vi "Configure IO Port.vi"(0 "VISA resource name":refnum<visa-resource-name>, 1 "Digital Output Pattern (1111)":u32=15 max=15 format="%04b", 2 "Enable I/O Port Auto Clear (F: Disable)":bool, 5 "Output Line 4 Mode (0: End of Test)":u16(ring) items=["End of Test", "Busy"], 7 "Active TTL Busy Level (0: Active Low)":u16(ring) items=["Active Low", "Active High"], 9 "Output Pattern Data Format (0: ASCII)":u16(ring) items=["ASCII", "Hexadecimal", "Octal", "Binary"], 11 "error in (no error)":errorcluster, 12 "Pass/Fail Pattern Delay (0.0001 s)":dbl=0.0001) -> (4 "VISA resource name out":refnum<visa-resource-name>, 15 "error out":errorcluster)   [LabVIEW 2020, in "Keithley 6517.lvlib"]
doc: "Configures the instrument's I/O port including the digital output clear pattern and Line 4 Mode.\n\n<B>Note:</B>\nThis VI is ONLY compatible with <B>model 6514</B>. Running this VI with any other model will result in an error."
uses:
  <instrlib>/Keithley 6517/Keithley 6517.lvlib
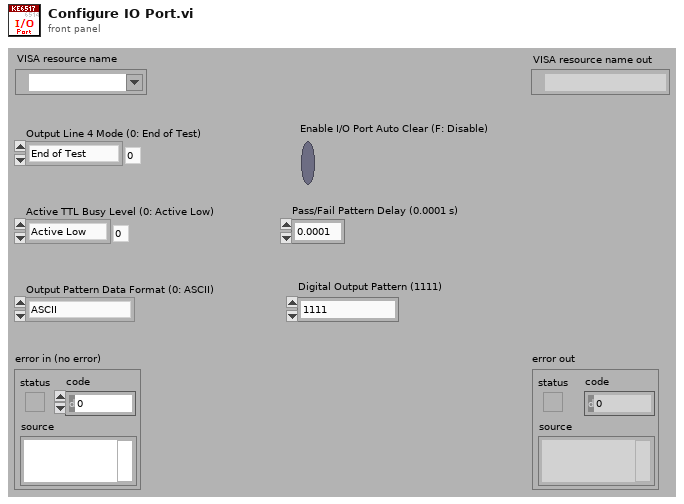
[diagram p1: front panel]
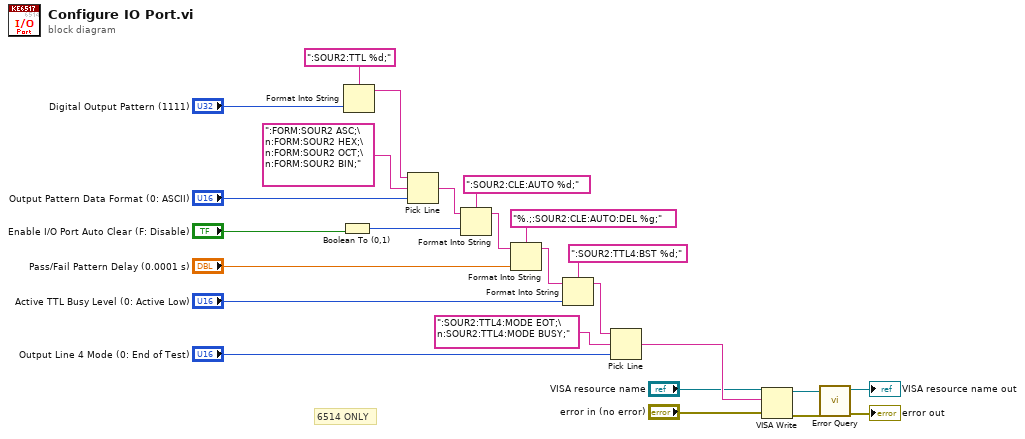
[diagram p0: block diagram]
diagram:
  # "6514 ONLY"
  n1 = Boolean To (0,1)(Boolean="Enable I/O Port Auto Clear (F: Disable)") -> (0, 1=w3:i16)
  n2 = Format Into String(format string=":SOUR2:TTL %d;", "Digital Output Pattern (1111)") -> (resulting string=w13:string)  [unwired: 2 in, 1 out]
  n3 = Pick Line(string ("")=w13, multi-line string=":FORM:SOUR2 ASC;\n:FORM:SOUR2 HEX;\n:FORM:SOUR2 OCT;\n:FORM:SOUR2 BIN;", line index="Output Pattern Data Format (0: ASCII)") -> (output string=w11:string)
  n4 = Format Into String(format string=":SOUR2:CLE:AUTO %d;", initial string=w11, w3) -> (resulting string=w9:string)  [unwired: 1 in, 1 out]
  n5 = Format Into String(format string="%.;:SOUR2:CLE:AUTO:DEL %g;", initial string=w9, "Pass/Fail Pattern Delay (0.0001 s)") -> (resulting string=w6:string)  [unwired: 1 in, 1 out]
  n6 = Format Into String(format string=":SOUR2:TTL4:BST %d;", initial string=w6, "Active TTL Busy Level (0: Active Low)") -> (resulting string=w5:string)  [unwired: 1 in, 1 out]
  n7 = Pick Line(string ("")=w5, multi-line string=":SOUR2:TTL4:MODE EOT;\n:SOUR2:TTL4:MODE BUSY;" ("format string"), line index="Output Line 4 Mode (0: End of Test)") -> (output string=w15:string)
  n8 = VISA Write(VISA resource name="VISA resource name", write buffer=w15, error in (no error)="error in (no error)") -> (VISA resource name out=w22:refnum<visa-resource-name>, error out=w23:errorcluster)  [unwired: 1 out]
  n9 = call <instrlib>:"Error Query.vi"("error in (no error)"=w23, "VISA resource name"=w22) -> ("error out"=→"error out":errorcluster, "VISA resource name out"=→"VISA resource name out":refnum<visa-resource-name>)  [unwired: 6 in, 2 out]
